vi "ExposeMapperSpliceNamepathToParts.vi"(11 "Namepath":string) -> (3 "Array of Strings":string[](array[string]))   [LabVIEW 2017]
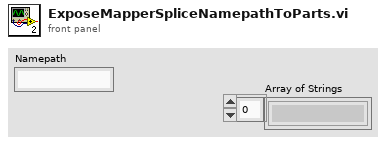
[diagram p1: front panel]
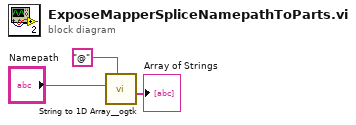
[diagram p0: block diagram]
diagram:
  n1 = call <userlib>:"String to 1D Array__ogtk.vi"("delimiter (Tab)"="@", "string"="Namepath") -> ("Array of Strings"=→"Array of Strings":string[])  [unwired: 9 in]
